vi "Publish Page.vi"(8 "error in (no error)":errorcluster {"code" format="Error %.0f"}, 9 "Publish Comment":string="Automated", 10 "Content":string, 11 "Page in":refnum<class "Page.lvclass">) -> (0 "error out":errorcluster {"code" format="Error %.0f"}, 1 "ID":string, 2 "Title":string, 3 "Page out":refnum<class "Page.lvclass">)   [LabVIEW 2023, in "VIDoc Printer - Confluence.lvlib" / "VIDoc Printer - Confluence.lvclass"]
uses:
  VIDoc Printer - Confluence.lvclass
  <userlib>/_PetranWay/LabVIEW Confluence API/Source/Confluence/Page/Page.lvclass
  <userlib>/_PetranWay/LabVIEW Confluence API/Source/Confluence/Page/Page.lvclass/Page.ctl
  <userlib>/_PetranWay/LabVIEW Confluence API/Source/Confluence/Page/Accessors/Write storage value.vi
  <userlib>/_PetranWay/LabVIEW Confluence API/Source/Confluence/Page/Accessors/Read title.vi
  <userlib>/_PetranWay/LabVIEW Confluence API/Source/Confluence/Page/Accessors/Read ID.vi
  <vilib>/JDP Science/JSONtext/Find Item.vi
  <userlib>/_PetranWay/LabVIEW Atlassian API/Source/JSON Utilities/Strip Quotes Around String.vi
  <vilib>/JDP Science/JSONtext/Next JSON Value.vi
  <vilib>/JDP Science/JSONtext/String Subset.vi
  <vilib>/JDP Science/JSONtext/Parsing/Advance past next JSON Value (inlined COPY).vi
  <vilib>/JDP Science/JSONtext/Parsing/Advance past whitespace.vi
  <vilib>/JDP Science/JSONtext/Parsing/Advance past String.vi
  <vilib>/JDP Science/JSONtext/Parsing/Advance past Number.vi
  <vilib>/JDP Science/JSONtext/Parsing/Advance past Line Ending.vi
  <vilib>/JDP Science/JSONtext/Parsing/Parse Full Path or Item Name.vi
  <vilib>/JDP Science/JSONtext/Parsing/Advance past Array.vi
  <vilib>/JDP Science/JSONtext/Parsing/Advance past Object.vi
  <vilib>/JDP Science/JSONtext/support/Error Cluster From Code.vi
  <vilib>/JDP Science/JSONtext/Offset/Find Item Locations by Path.vi
  <userlib>/_PetranWay/LabVIEW Confluence API/Source/Confluence/iConfluence/iConfluence.lvclass
  VIDoc Printer - Confluence.lvclass/VIDoc Printer - Confluence.ctl
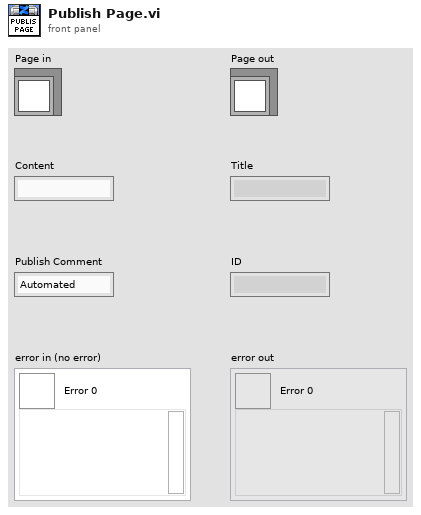
[diagram p1: front panel]
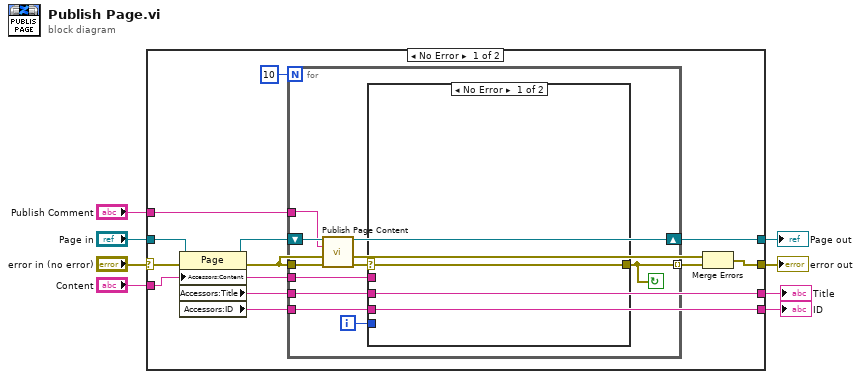
[diagram p0: block diagram]
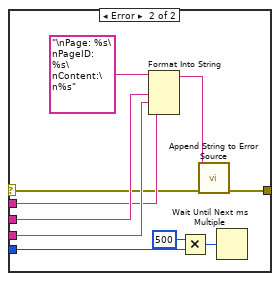
[diagram p2: hidden frame]
diagram:
  n1 = case shown="No Error" "error in (no error)" {
    selector: "error in (no error)" -> [w20 w43]
    tunnel: [w10 w43] -> w7
    tunnel: "Page in" -> [w11 w42]
    tunnel: [w15 w42] -> w5
    tunnel: "Publish Comment" -> [w17 _]
    tunnel: "Content" -> [w16 _]
    tunnel: [w14 _] -> w2
    tunnel: [w13 _] -> w1
    frame No Error {
      n2 = property class="Page"(reference=w11, error in=w20, "Accessors:Content"=w16) -> (reference out=w12:refnum<class "Page.lvclass">, error out=w9:errorcluster, "Accessors:Title"=w14:string, "Accessors:ID"=w13:string)
      n3 = for {
        N: 10 -> [_]
        tunnel: w17 -> [w28]
        shift-right: [w22] -> w15
        shift-left: w12 -> [w29]
        tunnel: w16 -> [w23]
        tunnel: w9 -> [w30]
        tunnel: [w26] -> w18 mode=indexing
        tunnel: w14 -> [w25]
        tunnel: w13 -> [w24]
        i -> [w21]
        stop <- w26 continue-if-true
        n4 = call-dynamic "Publish Page Content.vi"("Page"=w29, "Publish Comment"=w28, "error in (no error)"=w30) -> ("Page out"=w22:refnum<class "Page.lvclass">, "error out"=w27:errorcluster)  [unwired: 11 in]
        n5 = case shown="No Error" w27 {
          selector: w27 -> [w31 w37]
          tunnel: [w31 w36] -> w26
          tunnel: w25 -> [_ w40]
          tunnel: w24 -> [_ w39]
          tunnel: w23 -> [_ w38]
          tunnel: w21 -> [_ w34]
          frame No Error {
          }
          frame Error {
            n6 = Format Into String(format string="\nPage: %s\nPageID: %s\nContent:\n%s", w40, w39, w38) -> (resulting string=w35:string)  [unwired: 2 in, 1 out]
            n7 = Multiply(x=500, y=w34) -> (x*y=w33:i32)
            n8 = call "Append String to Error Source.vi"("Error In"=w37, "String to Append"=w35) -> ("Error Out"=w36:errorcluster)  [unwired: 9 in]
            n9 = Wait Until Next ms Multiple(millisecond multiple=w33) -> ()  [unwired: 1 out]
          }
        }
      }
      n10 = Merge Errors(w9, w18) -> (w10:errorcluster)
    }
    frame Error {
    }
  }
  "error out" <- w7
  "Page out" <- w5
  "Title" <- w2
  "ID" <- w1
